vi "SaveDeviceList.vi"(10 "DeviceList":T1(array[cluster]) {"Acquisition Parameters"."White level" scale=0.3..1.26 scale format="%#_2f"; "Acquisition Parameters"."Saturation" scale=0.5..1.5 scale format="%#_3f"; "Acquisition Parameters"."Contrast" scale=0.4..1.5 scale format="%#_3f"; "Acquisition Parameters"."Brightness" scale=-50.0..50.0 scale format="%#_2f"; "Correction Parameters"."Movement Type" items=["Step", "Proportionnal"]; "Target"."X Target" format="%#_5g"; "Target"."Y Target" format="%#_5g"; "Detection Parameters"."Max Intensity%" max=100 step=1}, 11 "path to XML document":path) -> (0 "error out":errorcluster, 3 "parse errors":string)   [LabVIEW 2013]
uses:
  <vilib>/xml/Load XML File.vi
  <resource>/objmgr/DOMUserDefRef.rc
  <vilib>/xml/NI_XML.lvlib
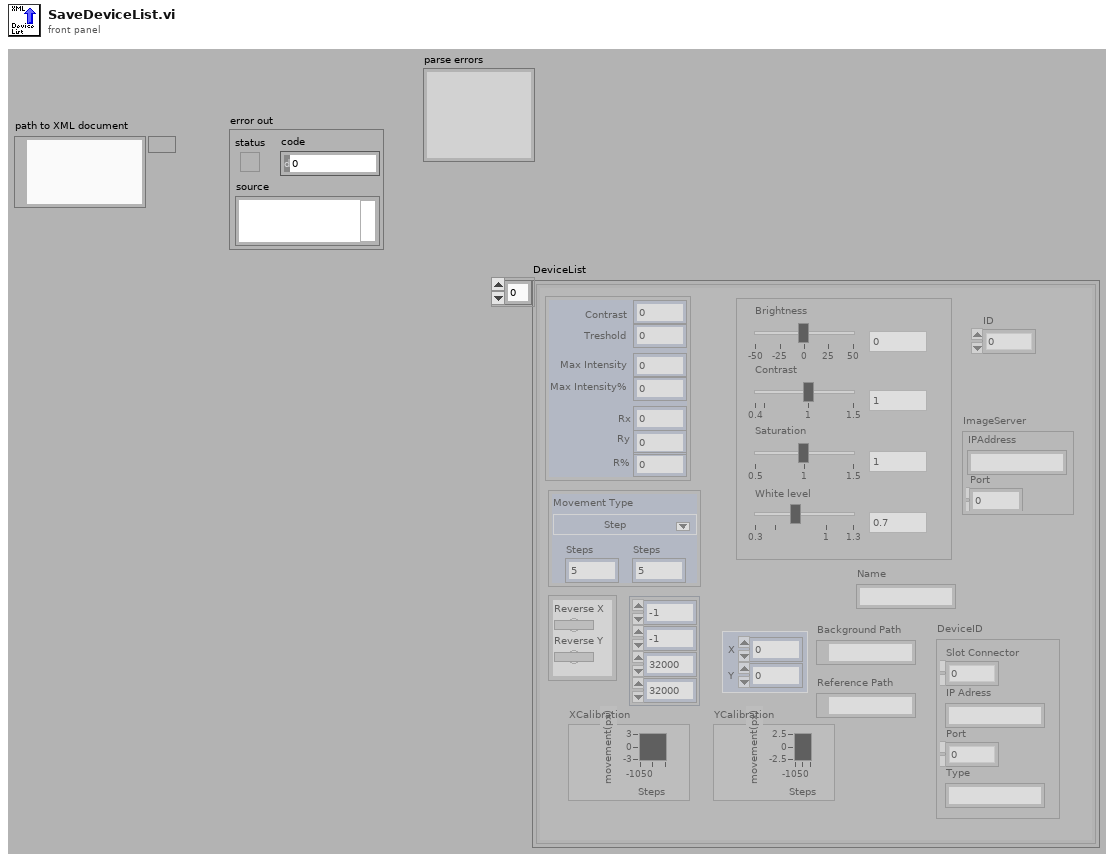
[diagram p1: front panel]
types:
  T1 = cluster{"ID":i32, "Name":string, "DeviceID":cluster{"Slot Connector":i32, "IP Adress":string, "Port":i32, "Type":string}, "Detection Parameters":cluster{"Contrast":i32, "Treshold":u8, "Max Intensity":i32, "Max Intensity%":u8, "Rx":i32, "Ry":i32, "R%":sgl}, "Reverse":cluster{"Reverse X":bool, "Reverse Y":bool}, "Target":cluster{"X Target":sgl, "Y Target":sgl}, "Region of Interest":i32[], "Correction Parameters":cluster{"X":sgl, "Y":sgl, "Movement Type":u16}, "Acquisition Parameters":cluster{"Brightness":dbl, "Contrast":dbl, "Saturation":dbl, "White level":dbl}, "Background Path":path, "Reference Path":path, "XCalibration":cluster{dbl, dbl}[], "YCalibration":cluster{dbl, dbl}[], "ImageServer":cluster{"IPAddress":string, "Port":i32}}[]
  T2 = cluster{"Slot Connector":i32, "IP Adress":string, "Port":i32, "Type":string}
  T3 = cluster{"Contrast":i32, "Treshold":u8, "Max Intensity":i32, "Max Intensity%":u8, "Rx":i32, "Ry":i32, "R%":sgl}
  T4 = cluster{"Brightness":dbl, "Contrast":dbl, "Saturation":dbl, "White level":dbl}
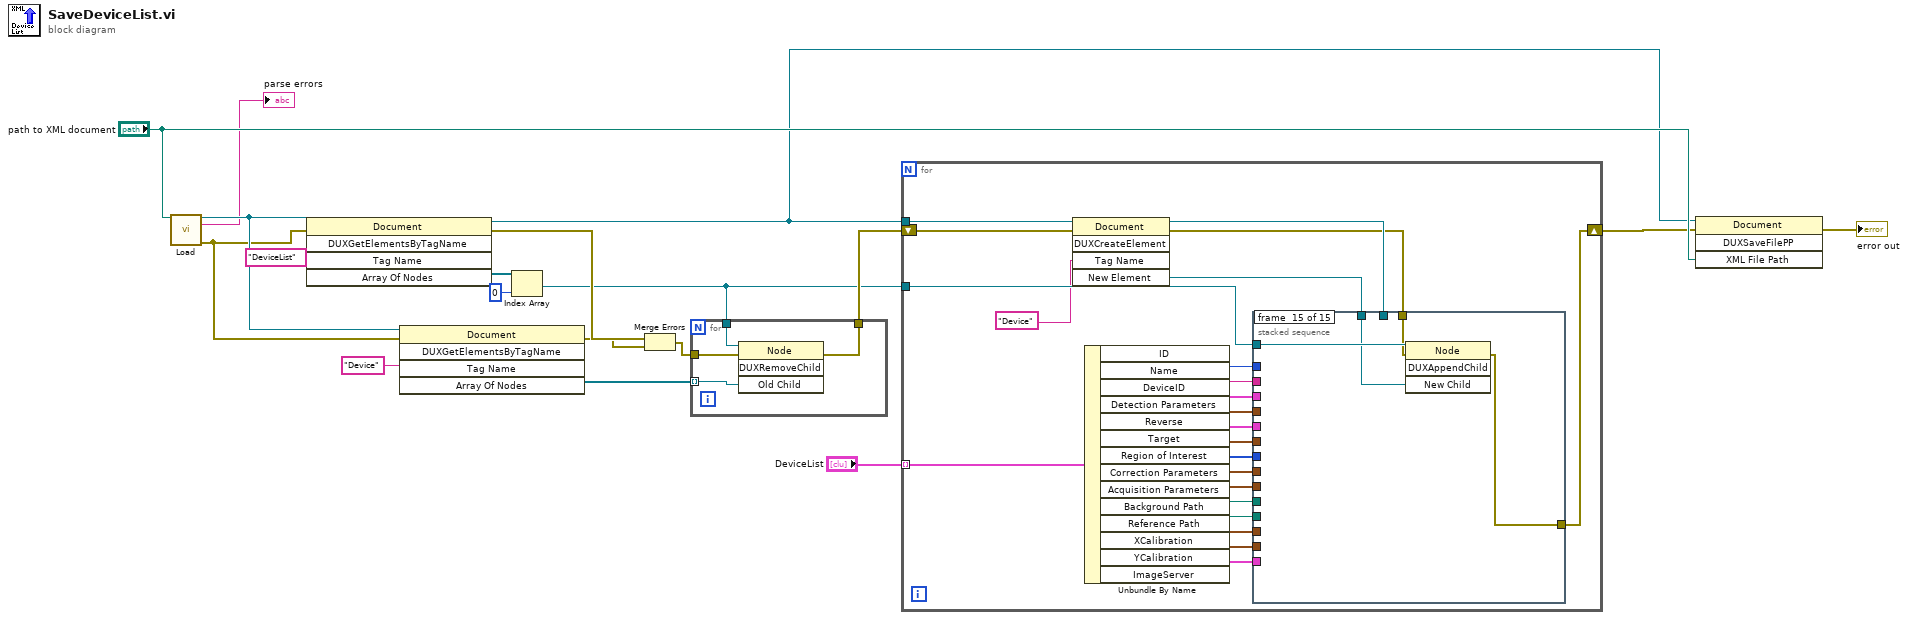
[diagram p0: block diagram]
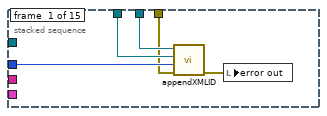
[diagram p2: hidden frame]
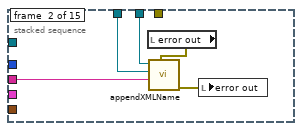
[diagram p3: hidden frame]
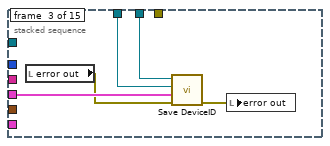
[diagram p4: hidden frame]
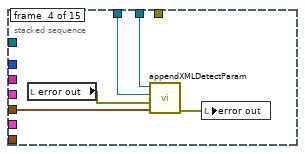
[diagram p5: hidden frame]
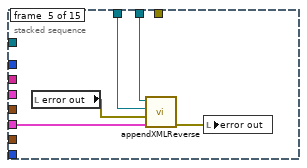
[diagram p6: hidden frame]
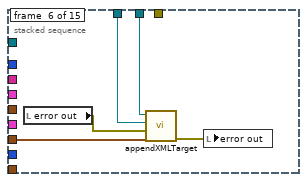
[diagram p7: hidden frame]
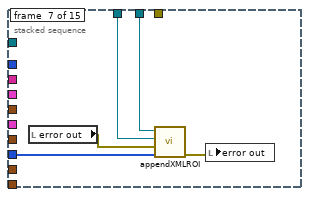
[diagram p8: hidden frame]
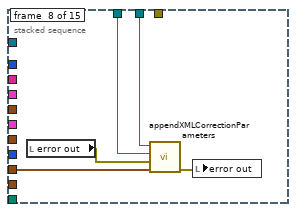
[diagram p9: hidden frame]
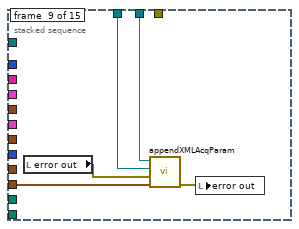
[diagram p10: hidden frame]
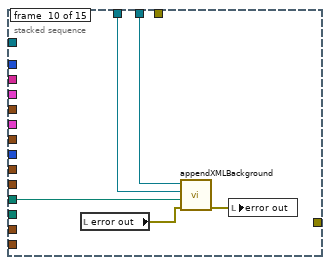
[diagram p11: hidden frame]
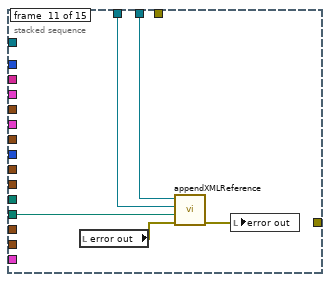
[diagram p12: hidden frame]
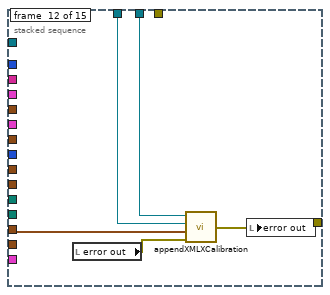
[diagram p13: hidden frame]
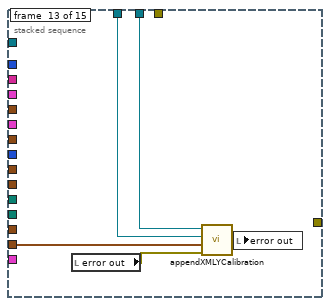
[diagram p14: hidden frame]
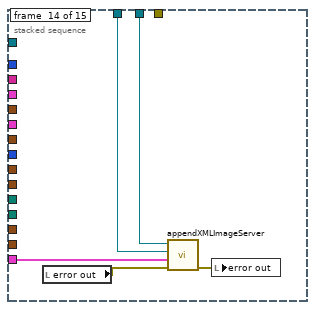
[diagram p15: hidden frame]
diagram:
  n1 = call-poly <vilib>:"Load.vi"("path to XML document"="path to XML document") -> ("DOM document out"=w15:refnum<k20>, "parse errors"=→"parse errors":string, "error out"=w13:errorcluster)  [unwired: 12 in]
  n2 = invoke class="Document" method="DUXGetElementsByTagName"(reference=w15, error in=w13, "Tag Name"="DeviceList") -> (reference out=w3:refnum<k20>, error out=w11:errorcluster, "Array Of Nodes"=w17:refnum<k20>[])  [unwired: 2 in, 2 out]
  n3 = invoke class="Document" method="DUXGetElementsByTagName"(reference=w15, error in=w13, "Tag Name"="Device") -> (error out=w10:errorcluster, "Array Of Nodes"=w14:refnum<k20>[])  [unwired: 2 in, 3 out]
  n4 = Index Array(array=w17, index=0) -> (element=w8:refnum<k20>)
  n5 = Merge Errors(w11, w10) -> (w12:errorcluster)
  n6 = for {
    tunnel: w8 -> [w22]
    tunnel: w14 -> [w21] mode=indexing
    tunnel: [w20] -> w9
    tunnel: w12 -> [w19]
    n7 = invoke class="Node" method="DUXRemoveChild"(reference=w22, error in=w19, "Old Child"=w21) -> (error out=w20:errorcluster)  [unwired: 1 in, 3 out]
  }
  n8 = for {
    tunnel: "DeviceList" -> [w44] mode=indexing
    tunnel: w3 -> [w45]
    tunnel: w8 -> [w31]
    shift-right: [w30] -> w2
    shift-left: w9 -> [w33]
    n9 = invoke class="Document" method="DUXCreateElement"(reference=w45, error in=w33, "Tag Name"="Device") -> (reference out=w34:refnum<k20>, error out=w32:errorcluster, "New Element"=w43:refnum<k20>)  [unwired: 2 in, 2 out]
    n10 = Unbundle By Name(w44) -> ("ID"=w26:i32, "Name"=w42:string, "DeviceID"=w41:T2, "Detection Parameters"=w40:T3, "Reverse"=w39:cluster{"Reverse X":bool, "Reverse Y":bool}, "Target"=w38:cluster{"X Target":sgl, "Y Target":sgl}, "Region of Interest"=w37:i32[], "Correction Parameters"=w36:cluster{"X":sgl, "Y":sgl, "Movement Type":u16}, "Acquisition Parameters"=w35:T4, "Background Path"=w29:path, "Reference Path"=w28:path, "XCalibration"=w25:cluster{dbl, dbl}[], "YCalibration"=w24:cluster{dbl, dbl}[], "ImageServer"=w23:cluster{"IPAddress":string, "Port":i32})
    n11 = stacked-sequence {
      tunnel: w43 -> [w49 w54 w59 w64 w69 w74 w79 w83 w88 w93 w99 w103 w108 w113 w118]
      tunnel: w34 -> [w50 w53 w60 w65 w70 w75 w80 w84 w89 w94 w100 w104 w109 w114 _]
      tunnel: w42 -> [_ w55 _ _ _ _ _ _ _ _ _ _ _ _ _]
      tunnel: w41 -> [_ _ w57 _ _ _ _ _ _ _ _ _ _ _ _]
      tunnel: w40 -> [_ _ _ w63 _ _ _ _ _ _ _ _ _ _ _]
      tunnel: w39 -> [_ _ _ _ w68 _ _ _ _ _ _ _ _ _ _]
      tunnel: w38 -> [_ _ _ _ _ w73 _ _ _ _ _ _ _ _ _]
      tunnel: w37 -> [_ _ _ _ _ _ w78 _ _ _ _ _ _ _ _]
      tunnel: w36 -> [_ _ _ _ _ _ _ w85 _ _ _ _ _ _ _]
      tunnel: w35 -> [_ _ _ _ _ _ _ _ w90 _ _ _ _ _ _]
      tunnel: w31 -> [_ _ _ _ _ _ _ _ _ _ _ _ _ _ w119]
      tunnel: w32 -> [w47 _ _ _ _ _ _ _ _ _ _ _ _ _ w117]
      tunnel: [_ _ _ _ _ _ _ _ _ _ _ _ _ _ w116] -> w30
      tunnel: w29 -> [_ _ _ _ _ _ _ _ _ w95 _ _ _ _ _]
      tunnel: w28 -> [_ _ _ _ _ _ _ _ _ _ w98 _ _ _ _]
      tunnel: w26 -> [w48 _ _ _ _ _ _ _ _ _ _ _ _ _ _]
      tunnel: w25 -> [_ _ _ _ _ _ _ _ _ _ _ w105 _ _ _]
      tunnel: w24 -> [_ _ _ _ _ _ _ _ _ _ _ _ w110 _ _]
      tunnel: w23 -> [_ _ _ _ _ _ _ _ _ _ _ _ _ w115 _]
      frame #0 {
        n12 = call "appendXMLID.vi"("error in (no error)"=w47, "ID"=w48, "Parent Device Node"=w49, "DOM document in"=w50) -> ("error out"=w46:errorcluster)  [unwired: 7 in]
        n13 = local write "error out"(w46) -> ()
      }
      frame #1 {
        n14 = local read "error out"() -> (w51:errorcluster)
        n15 = call "appendXMLName.vi"("error in (no error)"=w51, "name"=w55, "Parent Device Node"=w54, "DOM document in"=w53) -> ("error out"=w52:errorcluster)  [unwired: 7 in]
        n16 = local write "error out"(w52) -> ()
      }
      frame #2 {
        n17 = local read "error out"() -> (w56:errorcluster)
        n18 = call "Save DeviceID.vi"("error in (no error)"=w56, "DeviceID"=w57, "Parent Camera Node"=w59, "DOM document in"=w60) -> ("error out"=w58:errorcluster)  [unwired: 7 in]
        n19 = local write "error out"(w58) -> ()
      }
      frame #3 {
        n20 = local read "error out"() -> (w62:errorcluster)
        n21 = call "appendXMLDetectParam.vi"("Detection Parameters"=w63, "error in (no error)"=w62, "Parent Device Node"=w64, "DOM document in"=w65) -> ("error out"=w61:errorcluster)  [unwired: 7 in]
        n22 = local write "error out"(w61) -> ()
      }
      frame #4 {
        n23 = local read "error out"() -> (w66:errorcluster)
        n24 = call "appendXMLReverse.vi"("Reverse"=w68, "error in (no error)"=w66, "Parent Camera Node"=w69, "DOM document out"=w70) -> ("error out"=w67:errorcluster)  [unwired: 7 in]
        n25 = local write "error out"(w67) -> ()
      }
      frame #5 {
        n26 = local read "error out"() -> (w72:errorcluster)
        n27 = call "appendXMLTarget.vi"("Target"=w73, "error in (no error)"=w72, "Parent Camera Node"=w74, "DOM document in"=w75) -> ("error out"=w71:errorcluster)  [unwired: 7 in]
        n28 = local write "error out"(w71) -> ()
      }
      frame #6 {
        n29 = local read "error out"() -> (w77:errorcluster)
        n30 = call "appendXMLROI.vi"("DOM document in"=w80, "Parent Camera Node"=w79, "error in (no error)"=w77, "ROI"=w78) -> ("error out"=w76:errorcluster)  [unwired: 6 in]
        n31 = local write "error out"(w76) -> ()
      }
      frame #7 {
        n32 = local read "error out"() -> (w82:errorcluster)
        n33 = call "appendXMLCorrectionParameters.vi"("Correction Parameters"=w85, "error in (no error)"=w82, "Parent Camera Node"=w83, "DOM document in"=w84) -> ("error out"=w81:errorcluster)  [unwired: 7 in]
        n34 = local write "error out"(w81) -> ()
      }
      frame #8 {
        n35 = local read "error out"() -> (w87:errorcluster)
        n36 = call "appendXMLAcqParam.vi"("Acquisition Parameters"=w90, "error in (no error)"=w87, "Parent Camera Node"=w88, "DOM document in"=w89) -> ("error out"=w86:errorcluster)  [unwired: 7 in]
        n37 = local write "error out"(w86) -> ()
      }
      frame #9 {
        n38 = local read "error out"() -> (w92:errorcluster)
        n39 = call "appendXMLBackground.vi"("error in (no error)"=w92, "Background Path"=w95, "Parent Camera Node"=w93, "DOM document in"=w94) -> ("error out"=w91:errorcluster)  [unwired: 7 in]
        n40 = local write "error out"(w91) -> ()
      }
      frame #10 {
        n41 = local read "error out"() -> (w97:errorcluster)
        n42 = call "appendXMLReference.vi"("error in (no error)"=w97, "Reference Path"=w98, "Parent Camera Node"=w99, "DOM document in"=w100) -> ("error out"=w96:errorcluster)  [unwired: 7 in]
        n43 = local write "error out"(w96) -> ()
      }
      frame #11 {
        n44 = local read "error out"() -> (w101:errorcluster)
        n45 = call "appendXMLXCalibration.vi"("error in (no error)"=w101, "XCalibration"=w105, "Parent Device Node"=w103, "DOM document in"=w104) -> ("error out"=w102:errorcluster)  [unwired: 2 in]
        n46 = local write "error out"(w102) -> ()
      }
      frame #12 {
        n47 = local read "error out"() -> (w106:errorcluster)
        n48 = call "appendXMLYCalibration.vi"("error in (no error)"=w106, "YCalibration"=w110, "Parent Device Node"=w108, "DOM document in"=w109) -> ("error out"=w107:errorcluster)  [unwired: 2 in]
        n49 = local write "error out"(w107) -> ()
      }
      frame #13 {
        n50 = local read "error out"() -> (w112:errorcluster)
        n51 = call "appendXMLImageServer.vi"("error in (no error)"=w112, "ImageServer"=w115, "Parent Camera Node"=w113, "DOM document in"=w114) -> ("error out"=w111:errorcluster)  [unwired: 7 in]
        n52 = local write "error out"(w111) -> ()
      }
      frame #14 {
        n53 = invoke class="Node" method="DUXAppendChild"(reference=w119, error in=w117, "New Child"=w118) -> (error out=w116:errorcluster)  [unwired: 1 in, 3 out]
      }
    }
  }
  n54 = invoke class="Document" method="DUXSaveFilePP"(reference=w3, error in=w2, "XML File Path"="path to XML document") -> (error out=→"error out":errorcluster)  [unwired: 1 in, 3 out]
